vi "Test Resize.vi"() -> ()   [LabVIEW 2011]
uses:
  Tables/TBL2D.xctl
panel:
  in  "Stop Button":bool
  in  "TBL1D":cluster{"X":sgl[], "Y":sgl[], "Z":sgl[][]}(xcontrol)
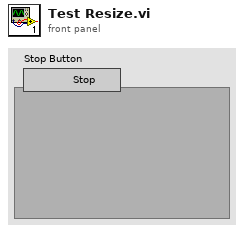
[diagram p1: front panel]
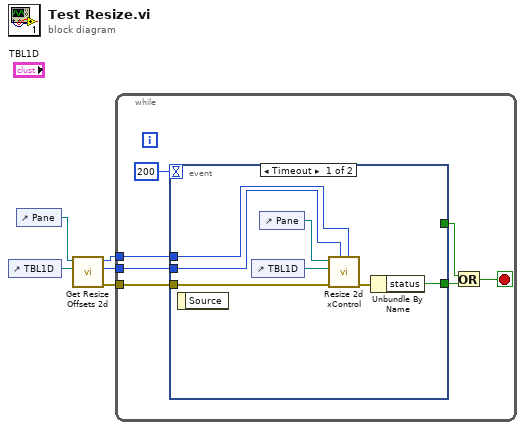
[diagram p0: block diagram]
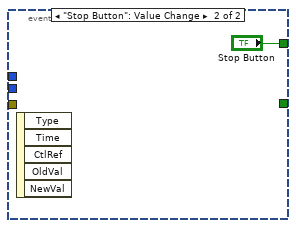
[diagram p2: hidden frame]
diagram:
  n1 = control-ref of="TBL1D"() -> (w1:refnum<vi>)
  n2 = control-ref of="Pane"() -> (w2:refnum<vi>)
  n3 = call "Get Resize Offsets 2d.vi"("TBL2D Refnum"=w1, "Pane in"=w2) -> ("error out"=w5:errorcluster, "Width Offset"=w3:u32, "Height Offset"=w4:u32)  [unwired: 7 in]
  n4 = while {
    tunnel: w5 -> [w10]
    tunnel: w4 -> [w7]
    tunnel: w3 -> [w6]
    stop <- w9 stop-if-true
    n5 = event shown="[0] Timeout" {
      selector: _ -> [_ _]
      dyn-events: _ -> [_ _]
      timeout: 200 -> [_ _]
      tunnel: [_ "Stop Button"] -> w12
      tunnel: w10 -> [w18 _]
      tunnel: [w19 _] -> w8
      tunnel: w7 -> [w15 _]
      tunnel: w6 -> [w16 _]
      event Timeout {
        n6 = event-data() -> ()  [unwired: 1 in, 1 out]
        n7 = control-ref of="TBL1D"() -> (w13:refnum<vi>)
        n8 = control-ref of="Pane"() -> (w14:refnum<vi>)
        n9 = call "Resize 2d xControl.vi"("Height Offset"=w15, "Width Offset"=w16, "error in (no error)"=w18, "Control in"=w13, "Pane"=w14) -> ("error out"=w17:errorcluster)  [unwired: 6 in]
        n10 = Unbundle By Name(w17) -> ("status"=w19:bool)
      }
      event "Stop Button": Value Change {
        n11 = event-data() -> ()  [unwired: 1 in, 5 out]
      }
    }
    n12 = Or(x=w12, y=w8) -> (x .or. y?=w9:bool)
  }
